vi "training_rating_display_sub.vi"(11 "Numeric":i32) -> (3 "Array 3":T1(array[cluster]))   [LabVIEW 2020]
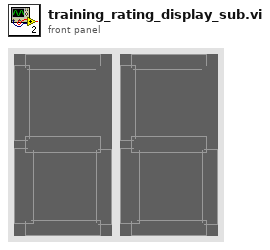
[diagram p1: front panel]
types:
  T1 = cluster{"Boolean":bool, "Boolean 2":bool, "Boolean 3":bool, "Boolean 4":bool, "Boolean 5":bool, "Boolean 6":bool, "Boolean 7":bool}[]
  T2 = cluster{"t[0]":bool, "t[1]":bool, "t[2]":bool, "t[3]":bool, "t[4]":bool, "t[5]":bool, "t[6]":bool}
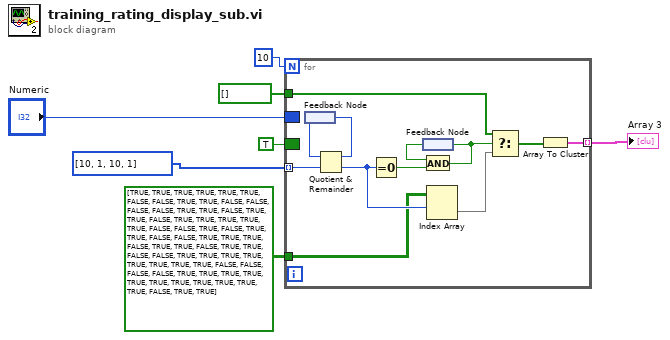
[diagram p0: block diagram]
diagram:
  n1 = for {
    N: 10 -> [_]
    border: "Numeric" -> [_]
    tunnel: i32[] [10, 1, 10, 1] -> [w17] mode=indexing
    tunnel: [w16] -> w1 mode=indexing
    border: TRUE -> [_]
    tunnel: bool[][] [[TRUE, TRUE, TRUE, TRUE, TRUE, TRUE, FALSE], [FALSE, TRUE, TRUE, FALSE, FALSE, FALSE, FALSE], [TRUE, TRUE, FALSE, TRUE, TRUE, FALSE, TRUE], [TRUE, TRUE, TRUE, TRUE, FALSE, FALSE, TRUE], [FALSE, TRUE, TRUE, FALSE, FALSE, TRUE, TRUE], [TRUE, FALSE, TRUE, TRUE, FALSE, TRUE, TRUE], [FALSE, FALSE, TRUE, TRUE, TRUE, TRUE, TRUE], [TRUE, TRUE, TRUE, FALSE, FALSE, FALSE, FALSE], [TRUE, TRUE, TRUE, TRUE, TRUE, TRUE, TRUE], [TRUE, TRUE, TRUE, TRUE, FALSE, TRUE, TRUE]] -> [w9]
    tunnel: bool[] [] ("t") -> [w8]
    n2 = feedback #1() -> (w18:i32)
    n3 = Quotient & Remainder(x=w18, y=w17) -> (x-y*floor(x/y)=w19:i32, floor(x/y)=w15:i32)
    n4 = feedback-in #1(w19) -> ()
    n5 = Equal To 0?(x=w15) -> (x = 0?=w14:bool)
    n6 = feedback #2() -> (w13:bool)
    n7 = And(x=w13, y=w14) -> (x .and. y?=w10:bool)
    n8 = feedback-in #2(w10) -> ()
    n9 = Index Array(array=w9, index (row)=w15) -> (element=w12:bool[])  [unwired: 1 in]
    n10 = Select(t=w8, s=w10, f=w12) -> (s? t:f=w11:bool[])
    n11 = Array To Cluster(array=w11) -> (cluster=w16:T2)
  }
  "Array 3" <- w1
